vi "Set Command Line.vi"(7 "environment variables":cluster{"name":string, "value":string}[](array[cluster]), 8 "error in (no error)":errorcluster, 9 "arguments":string[](array[string]), 10 "path":path, 11 "subprocess in":refnum<class "Subprocess.lvclass">) -> (0 "error out":errorcluster, 3 "subprocess out":refnum<class "Subprocess.lvclass">)   [LabVIEW 2020, in "NI_Subprocess.lvlib" / "Subprocess.lvclass"]
uses:
  <vilib>/Subprocess/Subprocess/Subprocess.lvclass
  <vilib>/Subprocess/Subprocess/Subprocess.lvclass/Subprocess.ctl
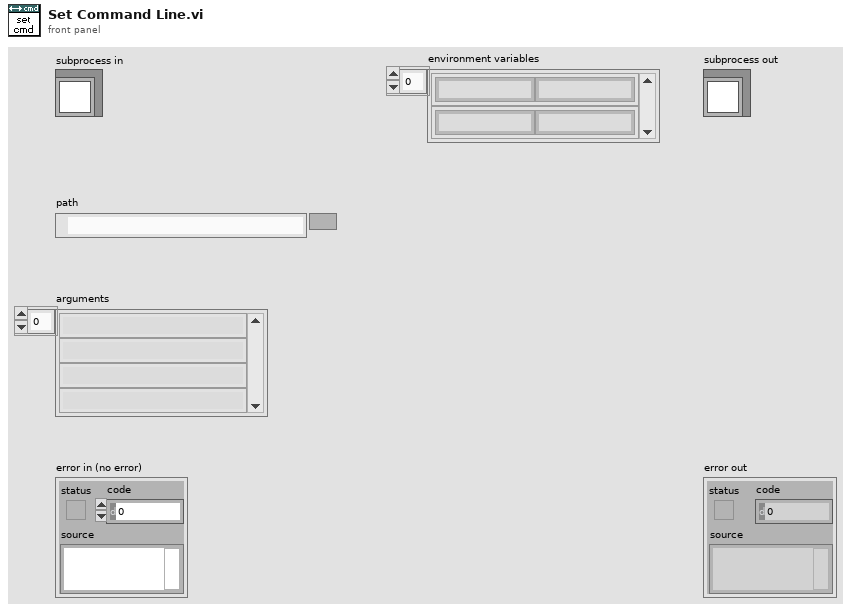
[diagram p1: front panel]
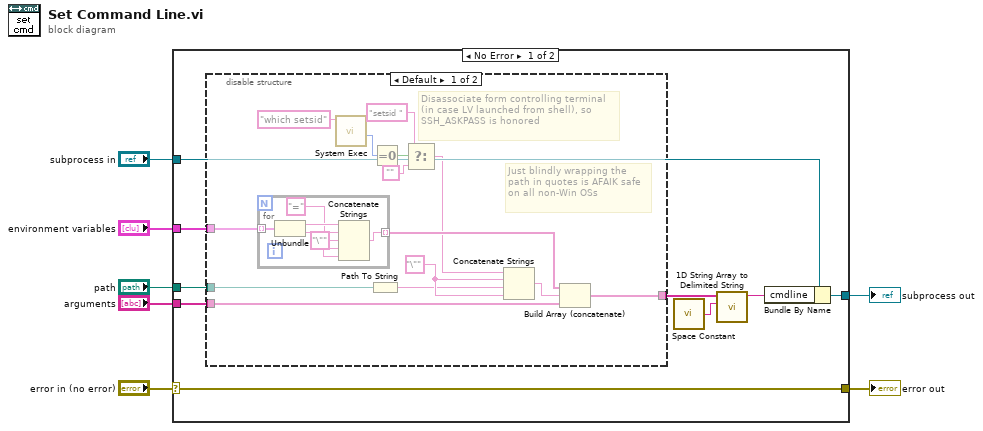
[diagram p0: block diagram]
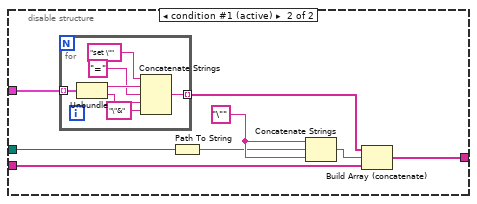
[diagram p2: hidden frame]
diagram:
  n1 = case shown="No Error" "error in (no error)" {
    selector: "error in (no error)" -> [w13 w53]
    tunnel: [w13 w53] -> w6
    tunnel: "path" -> [w16 _]
    tunnel: "arguments" -> [w15 _]
    tunnel: [w14 w52] -> w3
    tunnel: "subprocess in" -> [w9 w52]
    tunnel: "environment variables" -> [w8 _]
    frame No Error {
      n2 = disable-structure shown="Default" {
        disable-tunnel: w16 -> [w30 w44]
        disable-tunnel: w15 -> [w29 w43]
        disable-tunnel: [w28 w42] -> w11
        disable-tunnel: w8 -> [w27 w41]
        frame condition #0 {
          w25 = "\""
          # "Disassociate form controlling terminal (in case LV launched from shell), so SSH_ASKPASS is honored"
          # "Just blindly wrapping the path in quotes is AFAIK safe on all non-Win OSs"
          n3 = for {
            tunnel: w27 -> [w36] mode=indexing
            tunnel: [w32] -> w26 mode=indexing
            w31 = "\"" ("string")
            n4 = Unbundle(w36) -> ("name"=w35:string, "value"=w34:string)
            n5 = Concatenate Strings(w35, "=" ("string"), w31, w34, w31) -> (w32:string)
          }
          n6 = call <vilib>:"System Exec.vi"("command line"="which setsid") -> ("return code"=w21:i32)  [unwired: 7 in, 3 out]
          n7 = Path To String(path=w30) -> (string=w24:string)
          n8 = Equal To 0?(x=w21) -> (x = 0?=w20:bool)
          n9 = Select(t="setsid ", s=w20, f="") -> (s? t:f=w17:string)
          n10 = Concatenate Strings(w17, w25, w24, w25) -> (w23:string)
          n11 = Build Array (concatenate)(w26, w23, w29) -> (w28:string[])
        }
        frame condition #1 (active) {
          w39 = "\""
          n12 = for {
            tunnel: w41 -> [w51] mode=indexing
            tunnel: [w47] -> w40 mode=indexing
            n13 = Unbundle(w51) -> ("name"=w50:string, "value"=w49:string)
            n14 = Concatenate Strings("set \"" ("string"), w50, "=" ("string"), w49, "\"&" ("string")) -> (w47:string)
          }
          n15 = Path To String(path=w44) -> (string=w38:string)
          n16 = Concatenate Strings(w39, w38, w39) -> (w37:string)
          n17 = Build Array (concatenate)(w40, w37, w43) -> (w42:string[])
        }
      }
      n18 = call <vilib>:"Space Constant.vi"() -> ("String"=w12:string)
      n19 = call <vilib>:"1D String Array to Delimited String.vi"("delimiter"=w12, "string array"=w11) -> ("delimited string"=w10:string)  [unwired: 9 in]
      n20 = Bundle By Name(cluster=w9, "cmdline"=w10) -> (w14:refnum<class "Subprocess.lvclass">)
    }
    frame Error {
    }
  }
  "error out" <- w6
  "subprocess out" <- w3
